vi "Pressure Reads.vi"(8 "error in":errorcluster, 11 "Message Queues":T2) -> (0 "error out":errorcluster)   [LabVIEW 2021, in "Pressure.lvlib"]
uses:
  Pressure.lvlib
  <vilib>/DAQmx/create/channels.llb/DAQmx Create Channel (AI-Current-Basic).vi
  <vilib>/DAQmx/read.llb/DAQmx Read (Analog DBL 1Chan 1Samp).vi
  support/Message Queue/Enqueue Message (Single).vi
  support/Message Queue/Message Cluster.ctl
  support/Message Queue/All Message Queues.ctl
  support/Message Queue/Message Queue.lvlib
  PT Configuration.ctl
panel:
  in  "PT Configuration":T1={"physical channels"="cDAQ2Mod8/ai15", "name to assign"="Pressure", "units"=10342} {"units" items=["Amps"=10342, "From Custom Scale"=10065]}
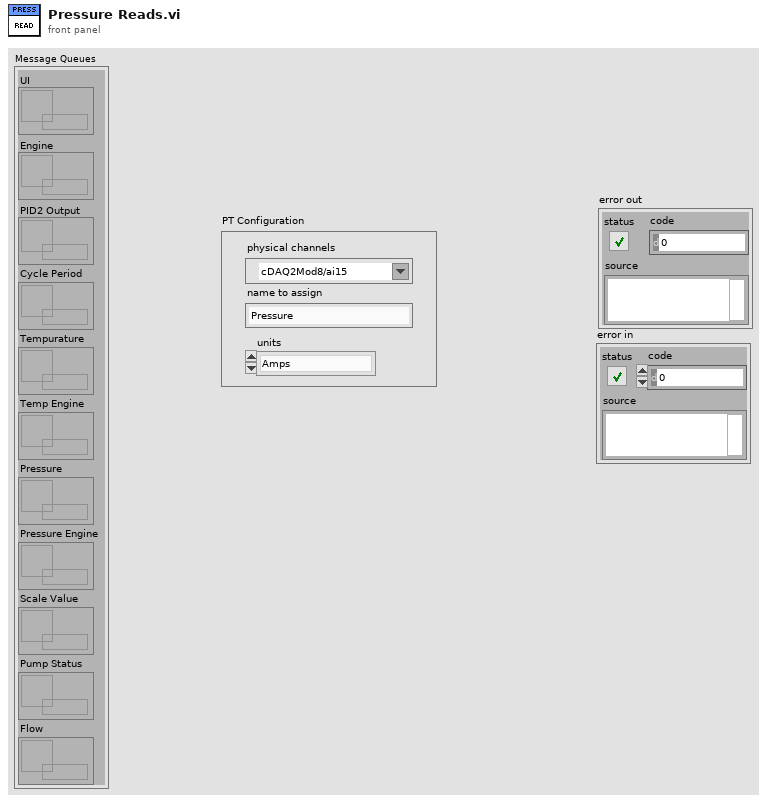
[diagram p1: front panel]
types:
  T1 = typedef "Pressure.lvlib/PT Configuration.ctl" = cluster{"physical channels":tag, "name to assign":string, "units":i32}
  T2 = typedef "Message Queue.lvlib/All Message Queues.ctl" = cluster{"UI":refnum<queue>, "Engine":refnum<queue>, "PID2 Output":refnum<queue>, "Cycle Period":refnum<queue>, "Tempurature":refnum<queue>, "Temp Engine":refnum<queue>, "Pressure":refnum<queue>, "Pressure Engine":refnum<queue>, "Scale Value":refnum<queue>, "Pump Status":refnum<queue>, "Flow":refnum<queue>}
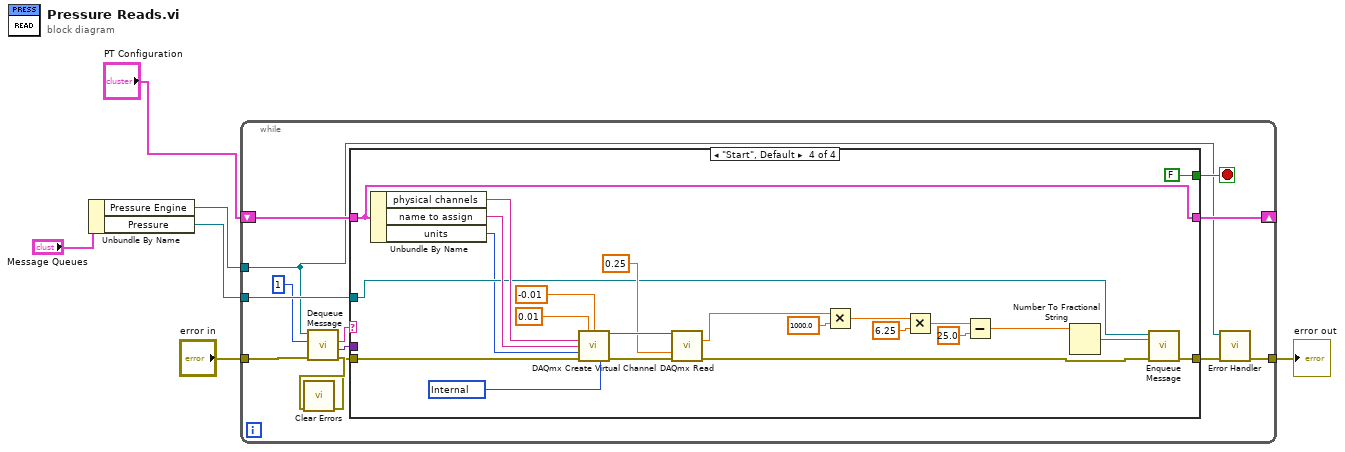
[diagram p0: block diagram]
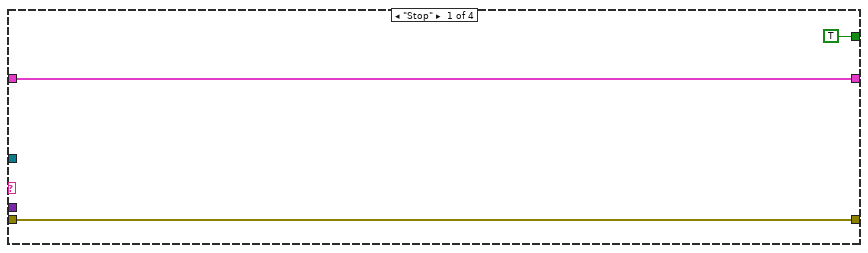
[diagram p2: hidden frame]
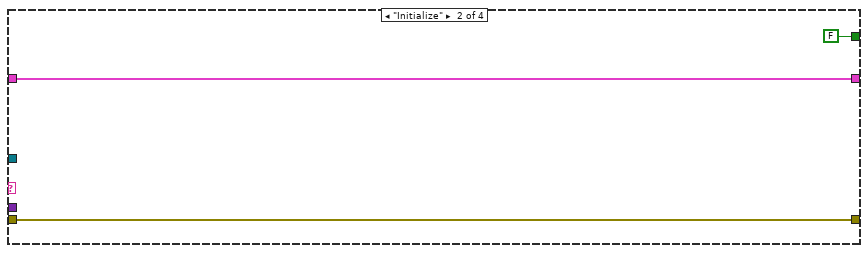
[diagram p3: hidden frame]
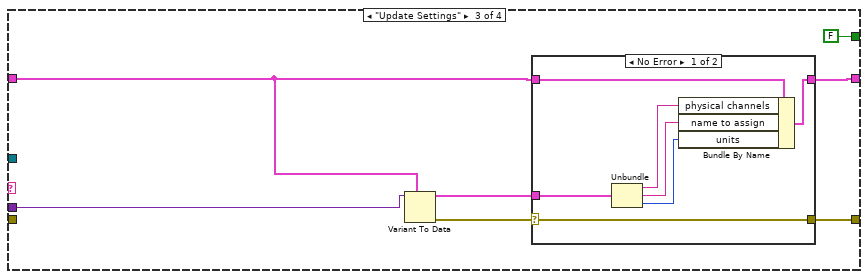
[diagram p4: hidden frame]
diagram:
  n1 = Unbundle By Name("Message Queues") -> ("Pressure Engine"=w3:refnum<queue>, "Pressure"=w2:refnum<queue>)
  n2 = while {
    tunnel: [w11] -> w5
    tunnel: w2 -> [w16]
    shift-right: [w18] -> _
    shift-left: "PT Configuration" -> [w17]
    tunnel: "error in" -> [w15]
    tunnel: w3 -> [w7]
    stop <- w19 stop-if-true
    n3 = call "Dequeue Message.vi"("error in (no error)"=w15, "timeout in ms (-1)"=1, "Message Queue"=w7) -> ("error out"=w9:errorcluster, "Message Data"=w14:variant, "Message"=w13:string)  [unwired: 5 in, 1 out]
    n4 = call <vilib>:"Clear Errors.vi"("error in (no error)"=w9) -> ("error out"=w8:errorcluster)  [unwired: 5 in, 1 out]
    n5 = case shown="\"Start\", Default" w13 {
      tunnel: w8 -> [w22 w24 _ w59]
      tunnel: [w22 w24 w29 w55] -> w12
      tunnel: [TRUE FALSE FALSE FALSE] -> w19
      tunnel: w16 -> [_ _ _ w57]
      tunnel: [w20 w25 w30 w54] -> w18
      tunnel: w17 -> [w20 w25 w26 w54]
      tunnel: w14 -> [_ _ w27 _]
      frame "Stop" {
      }
      frame "Initialize" {
      }
      frame "Update Settings" {
        n6 = Variant To Data(type=w26, Variant=w27) -> (data=w31:T1, error out=w32:errorcluster)  [unwired: 1 in]
        n7 = case shown="No Error" w32 {
          selector: w32 -> [w34 w40]
          tunnel: w26 -> [w39 w41]
          tunnel: w31 -> [w37 _]
          tunnel: [w38 w41] -> w30
          tunnel: [w34 w40] -> w29
          frame No Error {
            n8 = Unbundle(w37) -> ("physical channels"=w36:tag, "name to assign"=w35:string, "units"=w33:i32)
            n9 = Bundle By Name(cluster=w39, "physical channels"=w36, "name to assign"=w35, "units"=w33) -> (w38:T1)
          }
          frame Error {
          }
        }
      }
      frame "Start", Default {
        w50 = 10200 items=["default"=-1, "Internal"=10200, "External"=10167] ("shunt resistor location")
        n10 = Unbundle By Name(w54) -> ("physical channels"=w61:tag, "name to assign"=w60:string, "units"=w49:i32)
        n11 = call-poly <vilib>:"DAQmx Create Virtual Channel.vi"("maximum value"=0.01, "minimum value"=-0.01, "physical channels"=w61, "name to assign"=w60, "units"=w49, "error in"=w59, "shunt resistor location"=w50) -> ("task out"=w63:refnum<k21>, "error out"=w64:errorcluster)  [unwired: 7 in]
        n12 = call-poly <vilib>:"DAQmx Read.vi"("task/channels in"=w63, "timeout"=0.25, "error in"=w64) -> ("data"=w42:dbl, "error out"=w56:errorcluster)  [unwired: 10 in, 1 out]
        n13 = Multiply(x=w42, y=1000.0) -> (x*y=w45:dbl)
        n14 = Multiply(x=w45, y=6.25) -> (x*y=w46:dbl)
        n15 = Subtract(x=w46, y=25.0) -> (x-y=w43:dbl)
        n16 = Number To Fractional String(number=w43) -> (F-format string=w53:string)  [unwired: 3 in]
        n17 = call-poly "Enqueue Message.vi"("error in (no error)"=w56, "Message"=w53, "Message Queue"=w57) -> ("error out"=w55:errorcluster)  [unwired: 7 in, 1 out]
      }
    }
    n18 = call "Error Handler.vi"("error in (no error)"=w12, "Message Queue"=w7) -> ("dup error in"=w11:errorcluster)  [unwired: 8 in, 1 out]
  }
  "error out" <- w5
